vi "Test_HelloWorld_InvalidAsciiEncoding.vi"() -> (0 "Array of Error Description":T1)   [LabVIEW 2019]
uses:
  gRPC_ATS/TestUtility/utility.llb/array of error description.ctl
  gRPC_ATS/TestUtility/utility.llb/error description.ctl
  gRPC_ATS/TestUtility/utility.llb/error type.ctl
  examples/helloworld/helloworld_client/RPC Messages/helloworld_HelloRequest.ctl
  690210b7-9fc1-4805-899f-f09b8e1640af.vi
  <vilib>/gRPC/LabVIEW gRPC Library/Server API/Translate Protobuf Error.vi
  <vilib>/AdvancedString/1D String Array to Delimited String.vi
  <vilib>/gRPC/LabVIEW gRPC Library/Server API/Server/Get Server DLL Path.vi
  examples/helloworld/helloworld_client/helloworld_client.lvlib
panel:
  out "Pass":bool
  in  "error in (no error)":errorcluster
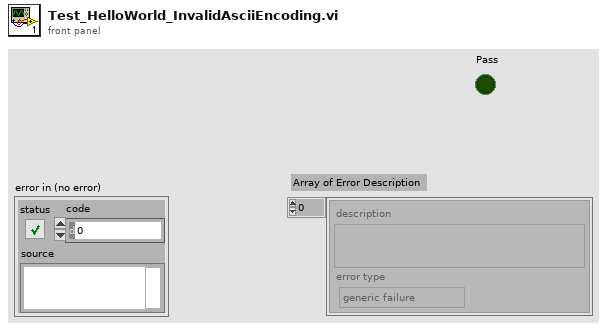
[diagram p1: front panel]
types:
  T1 = typedef "array of error description.ctl" = T2[]
  T2 = typedef "error description.ctl" = cluster{"description":string, "error type":T3}
  T3 = typedef "error type.ctl" = enum32{"generic failure", "boundary case", "precision", "expected error"}
  T4 = typedef "helloworld_client.lvlib/helloworld_HelloRequest.ctl" = cluster{"name":string}
  T5 = typedef "grpc-lvsupport-release.lvlib/grpcId.ctl" = u64
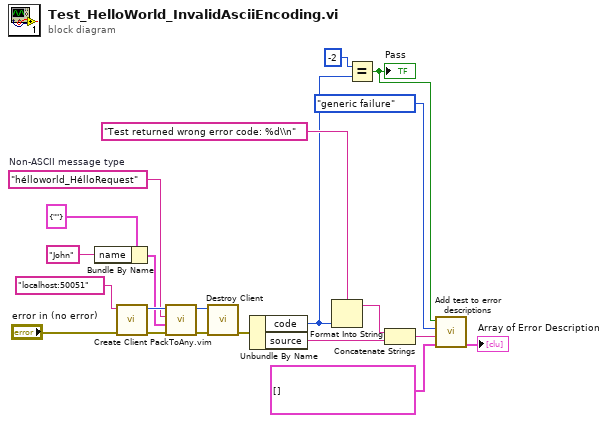
[diagram p0: block diagram]
diagram:
  w11 = "hélloworld_HélloRequest"  # Non-ASCII message type
  n1 = Bundle By Name(cluster=T4 {"name"=""} ("helloworld_HelloRequest"), "name"="John") -> (w12:T4)
  n2 = call "Create Client.vi"("error in"="error in (no error)", "address"="localhost:50051") -> ("error out"=w16:errorcluster, "gRPC ID Out"=w15:T5)  [unwired: 8 in]
  n3 = call "PackToAny.vim"("error in"=w16, "Data To Pack"=w12, "Message Type"=w11, "gRPCid in"=w15) -> ("error out"=w5:errorcluster, "gRPCid out"=w8:u64)  [unwired: 5 in, 1 out]
  n4 = call "Destroy Client.vi"("error in"=w5, "gRPC ID"=w8) -> ("error out"=w9:errorcluster)  [unwired: 9 in]
  n5 = Unbundle By Name(w9) -> ("code"=w2:i32, "source"=w18:string)
  n6 = Format Into String(format string="Test returned wrong error code: %d\\n" ("string"), w2) -> (resulting string=w1:string)  [unwired: 2 in, 1 out]
  n7 = Equal?(x=-2, y=w2) -> (x = y?=w6:bool)
  "Pass" <- w6
  n8 = Concatenate Strings(w1, w18) -> (w19:string)
  n9 = call "Add test to error descriptions.vi"("error descriptions in"=T1 [], "error string"=w19, "error type"=error_type."generic failure", "pass"=w6) -> ("error description out"=→"Array of Error Description":T1)  [unwired: 3 in]
